vi "Is Locked.vi"(8 "error in":errorcluster) -> (0 "error out":errorcluster, 3 "Locked?":bool)   [LabVIEW 2016, in "Drive System.lvlib"]
uses:
  Drive System.lvlib
  Private/Raw Data.vi
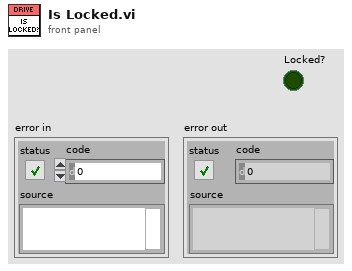
[diagram p1: front panel]
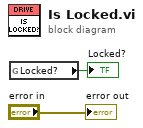
[diagram p0: block diagram]
diagram:
  n1 = global read "Raw Data.vi" "Locked?"() -> (→"Locked?":bool)
  "error out" <- "error in"
